vi "CleanupHumidityData.vi"(1 "HygrostatData":dbl[](array[numeric]), 2 "Data Return In":string[](array[string])) -> (0 "Data Return Out":string[](array[string]))   [LabVIEW 2024]
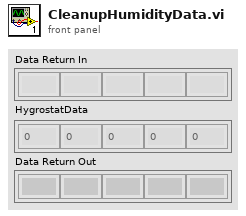
[diagram p1: front panel]
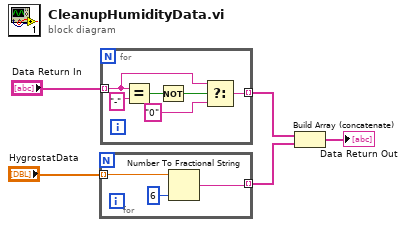
[diagram p0: block diagram]
diagram:
  n1 = for {
    tunnel: "HygrostatData" -> [w8] mode=indexing
    tunnel: [w7] -> w3 mode=indexing
    n2 = Number To Fractional String(number=w8, precision (6)=i16 6) -> (F-format string=w7:string)  [unwired: 2 in]
  }
  n3 = for {
    tunnel: "Data Return In" -> [w11] mode=indexing
    tunnel: [w9] -> w2 mode=indexing
    n4 = Equal?(x=w11, y="-") -> (x = y?=w13:bool)
    n5 = Not(x=w13) -> (.not. x?=w12:bool)
    n6 = Select(t=w11, s=w12, f="0" ("t")) -> (s? t:f=w9:string)
  }
  n7 = Build Array (concatenate)(w2, w3) -> (→"Data Return Out":string[])
